vi "format set font script.vi"(8 "error in (no error)":errorcluster, 10 "style":u8, 11 "format":u32) -> (0 "error out":errorcluster)   [LabVIEW 2015, in "xlsxwriter.lvlib"]
doc: "void format_set_font_script(lxw_format format, uint8_t style);"
uses:
  xlsxwriter.lvlib
  xlsxwriter.dll
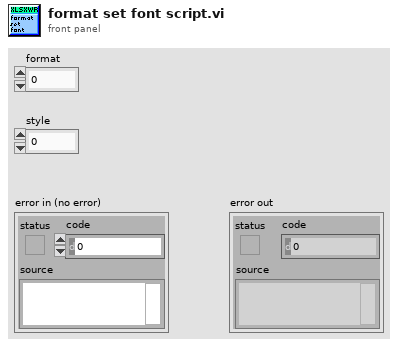
[diagram p1: front panel]
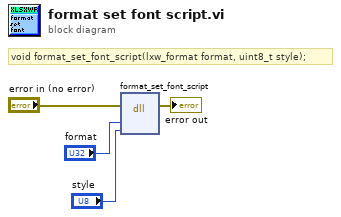
[diagram p0: block diagram]
diagram:
  # "void format_set_font_script(lxw_format format, uint8_t style);"
  n1 = dll-call lib="C:/Users/WDAGUtilityAccount/Desktop/lv_vis_added_cell/xlsxwriter.*" fn="format_set_font_script"(error in="error in (no error)", "format"="format", "style"="style") -> (error out=→"error out":errorcluster)  [unwired: 5 in, 1 out]
